vi "sub UI set o.vi"(8 "error in (no error)":errorcluster, 10 "<o> data":T1, 11 "IDE simple in":refnum<class "LF2R IDE.lvclass">) -> (0 "error out":errorcluster, 3 "IDE simple out":refnum<class "LF2R IDE.lvclass">)   [LabVIEW 2018, in "LF2R IDE.lvlib" / "LF2R IDE.lvclass"]
uses:
  LF2R IDE.lvclass
  Frame Analizer/frame o data.ctl
  LF2R IDE.lvclass/LF2R IDE.ctl
  Frame Analizer/Data Parser.lvclass
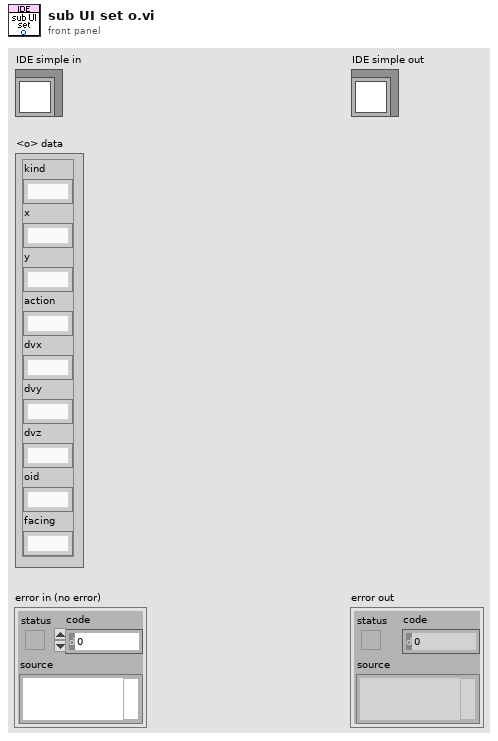
[diagram p1: front panel]
types:
  T1 = typedef "Data Parser.lvclass/frame o data.ctl" = cluster{"kind":string, "x":string, "y":string, "action":string, "dvx":string, "dvy":string, "dvz":string, "oid":string, "facing":string}
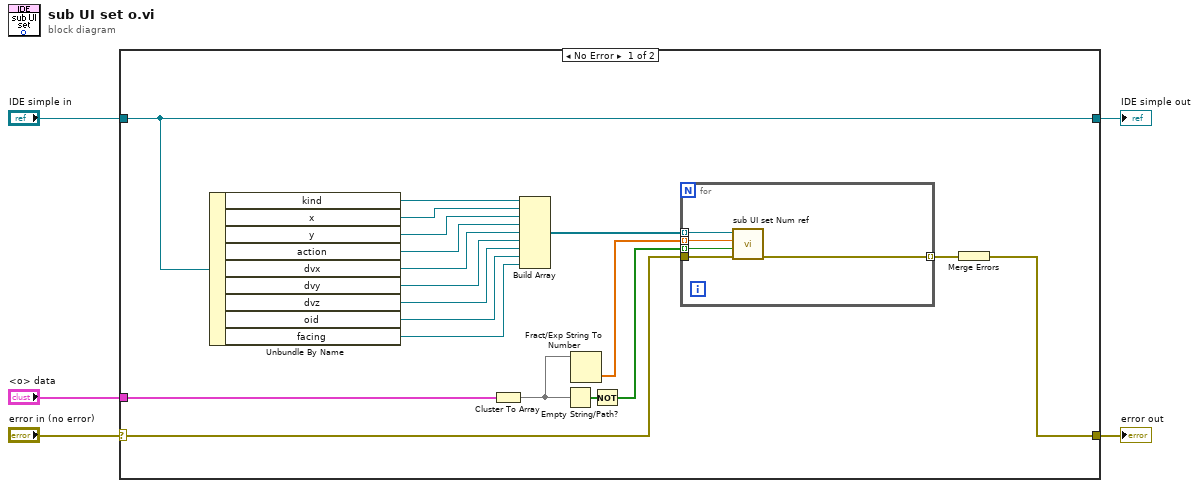
[diagram p0: block diagram]
diagram:
  n1 = case shown="No Error" "error in (no error)" {
    selector: "error in (no error)" -> [w23 w31]
    tunnel: [w18 w31] -> w4
    tunnel: [w20 w30] -> w2
    tunnel: "IDE simple in" -> [w20 w30]
    tunnel: "<o> data" -> [w17 _]
    frame No Error {
      n2 = Unbundle By Name(w20) -> ("kind"=w14:refnum<vi>, "x"=w13:refnum<vi>, "y"=w12:refnum<vi>, "action"=w11:refnum<vi>, "dvx"=w10:refnum<vi>, "dvy"=w9:refnum<vi>, "dvz"=w8:refnum<vi>, "oid"=w7:refnum<vi>, "facing"=w6:refnum<vi>)
      n3 = Cluster To Array(cluster=w17) -> (array=w16:string[])
      n4 = Build Array(w14, w13, w12, w11, w10, w9, w8, w7, w6) -> (w15:refnum<vi>[])
      n5 = Empty String/Path?(string/path=w16) -> (empty?=w24:bool[])
      n6 = Fract/Exp String To Number(string=w16) -> (number=w21:dbl[])  [unwired: 3 in, 1 out]
      n7 = Not(x=w24) -> (.not. x?=w22:bool[])
      n8 = for {
        tunnel: w23 -> [w29]
        tunnel: w15 -> [w25] mode=indexing
        tunnel: w22 -> [w26] mode=indexing
        tunnel: w21 -> [w28] mode=indexing
        tunnel: [w27] -> w19 mode=indexing
        n9 = call "sub UI set Num ref.vi"("error in"=w29, "valid"=w26, "Value"=w28, "num ref"=w25) -> ("error out"=w27:errorcluster)  [unwired: 7 in]
      }
      n10 = Merge Errors(w19) -> (w18:errorcluster)
    }
    frame Error {
    }
  }
  "error out" <- w4
  "IDE simple out" <- w2
